vi "Timeout Selector.vi"(6 "Remaining States":string, 7 "Timeout Expected":i32) -> (3 "Timeout":i32)   [LabVIEW 2020, in "Communicable State Machine.lvlib"]
doc: "Used in User Event Template VI.\n\n<b>Inputs:</b>\n - <b>Timeout Expected</b>: Expected timeout\n - <b>Remaining States</b>: If any remaining states left, output will be 0, otherwise, output is the expected value.\n\n<b>Outputs:</b>\n - <b>Timeout</b>: timeout will be used."
uses:
  Communicable State Machine.lvlib
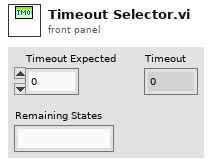
[diagram p1: front panel]
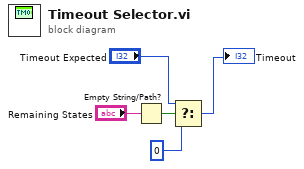
[diagram p0: block diagram]
diagram:
  n1 = Empty String/Path?(string/path="Remaining States") -> (empty?=w2:bool)
  n2 = Select(t="Timeout Expected", s=w2, f=0) -> (s? t:f=→"Timeout":i32)
